vi "MainProgram.vi"() -> ()   [LabVIEW 2018]
uses:
  GitLabRepo/testers_labview/Library/Colas/FGV Control App Station.ctl
  GitLabRepo/testers_labview/ControlsApps/QueueLastState.ctl
  GitLabRepo/testers_labview/ControlsApps/ActionFGVConfig.ctl
  GitLabRepo/testers_labview/Library/NI/AMC_Klagan/Read Termination Message.vi
  GitLabRepo/testers_labview/Library/NI/AMC_Klagan/Create Single Message.vi
  GitLabRepo/testers_labview/Library/NI/AMC_Klagan/Update Message Routing Info.vi
  GitLabRepo/testers_labview/Library/NI/AMC_Klagan/Send Message.vi
  GitLabRepo/testers_labview/Library/NI/AMC_Klagan/Globals.vi
  GitLabRepo/testers_labview/Library/NI/AMC_Klagan/Queue Registry.vi
  <vilib>/Utility/file.llb/Write Delimited Spreadsheet (DBL).vi
  GitLabRepo/testers_labview/Library/NI/AMC_Klagan/AMC_Klagan.lvlib
panel:
  in  "ReadAnalogInputs":bool
  out "Out 7":bool
  out "Out 6":bool
  out "Out 5":bool
  out "Out 4":bool
  out "Out 3":bool
  out "Out 2":bool
  in  "WU_CreateUser":bool
  in  "WU_EditUser":bool
  in  "WU_RemoveUser":bool
  in  "WU_Role":enum16{"Manager", "Technician", "Operator"}(ring)=enum."Operator" caption="Role"
  in  "error in":errorcluster
  in  "Window":string
  # "ARDUINO UNO"
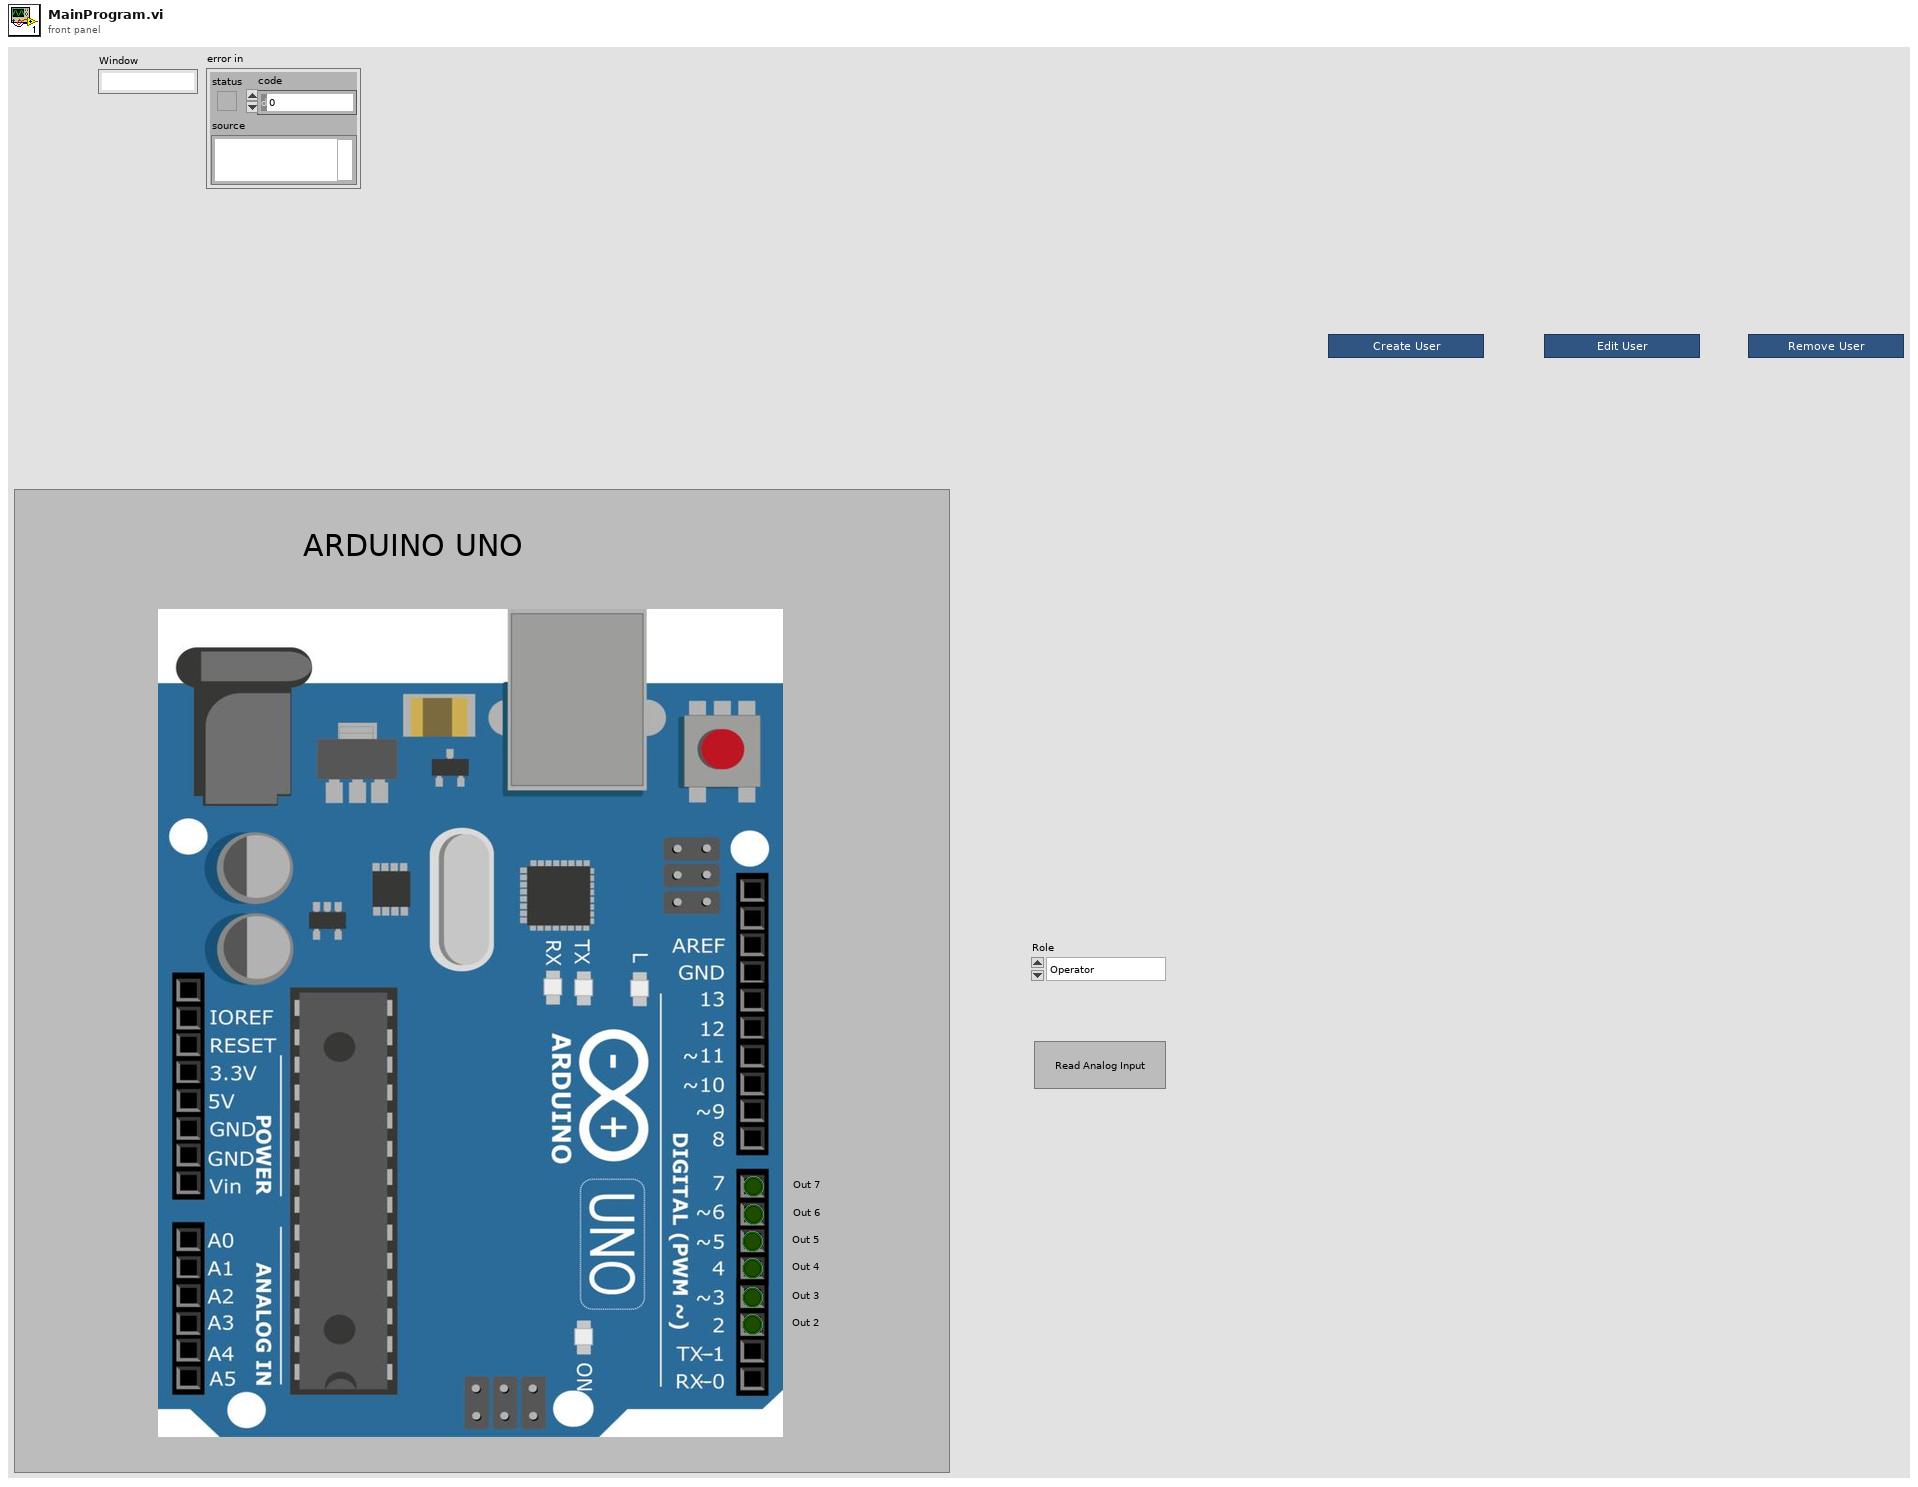
[diagram p1: front panel]
types:
  T1 = typedef "QueueLastState.ctl" = cluster{"LastState":string, "Data":variant}
  T2 = typedef "FGV Control App Station.ctl" = enum16{"Set", "Get All", "RemoveQueue", "Init"}
  T3 = typedef "AMC_Klagan.lvlib/Message Queue.ctl" = refnum<queue>
  T4 = typedef "ActionFGVConfig.ctl" = enum16{"SaveConfig", "ReadConfig"}
  T5 = typedef "GeneralConfig.ctl" = cluster{"General":path, "Path_Plataforma":path, "Path_Save_Sequences":path, "Path_Debugger":path, "Path_Logs_Tests":path, "Path_Reports":path, "Name_Station":string, "Path_Tests":path, "Path_Icons":path, "NumberOfCells":u32, "Path_TemplateReport":path, "Path_PowerUp":path, "Path_PowerDown":path, "Path_Abort":path, "Path_StartSequence":path, "Path_FinisSequence":path, "PortServerAPP":u32, "Path_Logs_App":path, "ExecutionDefSeqWhenOpen":bool, "LoadDefSeqWhenOpen":bool, "DefaultSequences":T6, "EnableSaveReports":bool, "EnableLogSequence":bool, "EnableDebuggerFile":bool, "Path_DefaultSequenceStart":path, "Path_DefaultSequenceAbort":path, "ManagerCommunication":T7, "Path_Factory":path, "Path_Variant":path, "Path_Model":path, "Path_SaveConfig":path, "SelectINI":string, "Path_ConfigPinOut":path, "Path_FailSequence":path, "Path_FinishExecutionSequence":path, "Path_DefaultSeqPowerUp":path, "Path_DefaultSeqPowerDown":path, "Path_DefaultSeqFinish":path, "Path_DefaultSeqFail":path, "Path_DefaultFinishExecution":path, "EnablePowerUpWhenOpen":bool, "EnablePowerDownWhenClose":bool, "EnableFinishExecution":bool, "SimultaneousStartCell":bool, "DefaultSimultaneousStartCellExecuteContinuously":bool, "DefaultHiddenStartSeq":bool, "DefaultHiddenAbortSeq":bool, "DefaultHiddenFinishExec":bool, "DefaultHiddenFailSeq":bool, "DefaultHiddenFinishSeq":bool, "DefaultHiddenPowerDown":bool, "DefaultHiddenPowerUp":bool, "Path_Users":path, "Path_File_Translate":path, "Path Icon 1":path, "Path Icon 2":path, "Path Image Login":path, "Check PCName Vs StationName":bool, "Windows Cells Layout":string, "Only One Test Plan for all cells":bool}
  T6 = typedef "DefaultSequncesLoad.ctl" = cluster{"Path_DefaultSeqCell 1":path, "Path_DefaultSeqCell 2":path, "Path_DefaultSeqCell 3":path, "Path_DefaultSeqCell 4":path, "Path_DefaultSeqCell 5":path, "Path_DefaultSeqCell 6":path, "Path_DefaultSeqCell 7":path, "Path_DefaultSeqCell 8":path, "Path_DefaultSeqCell 9":path}
  T7 = typedef "ConfiManagerCommunication.ctl" = cluster{"PortManComm":u32, "IPManager":string, "EnableManCom":bool}
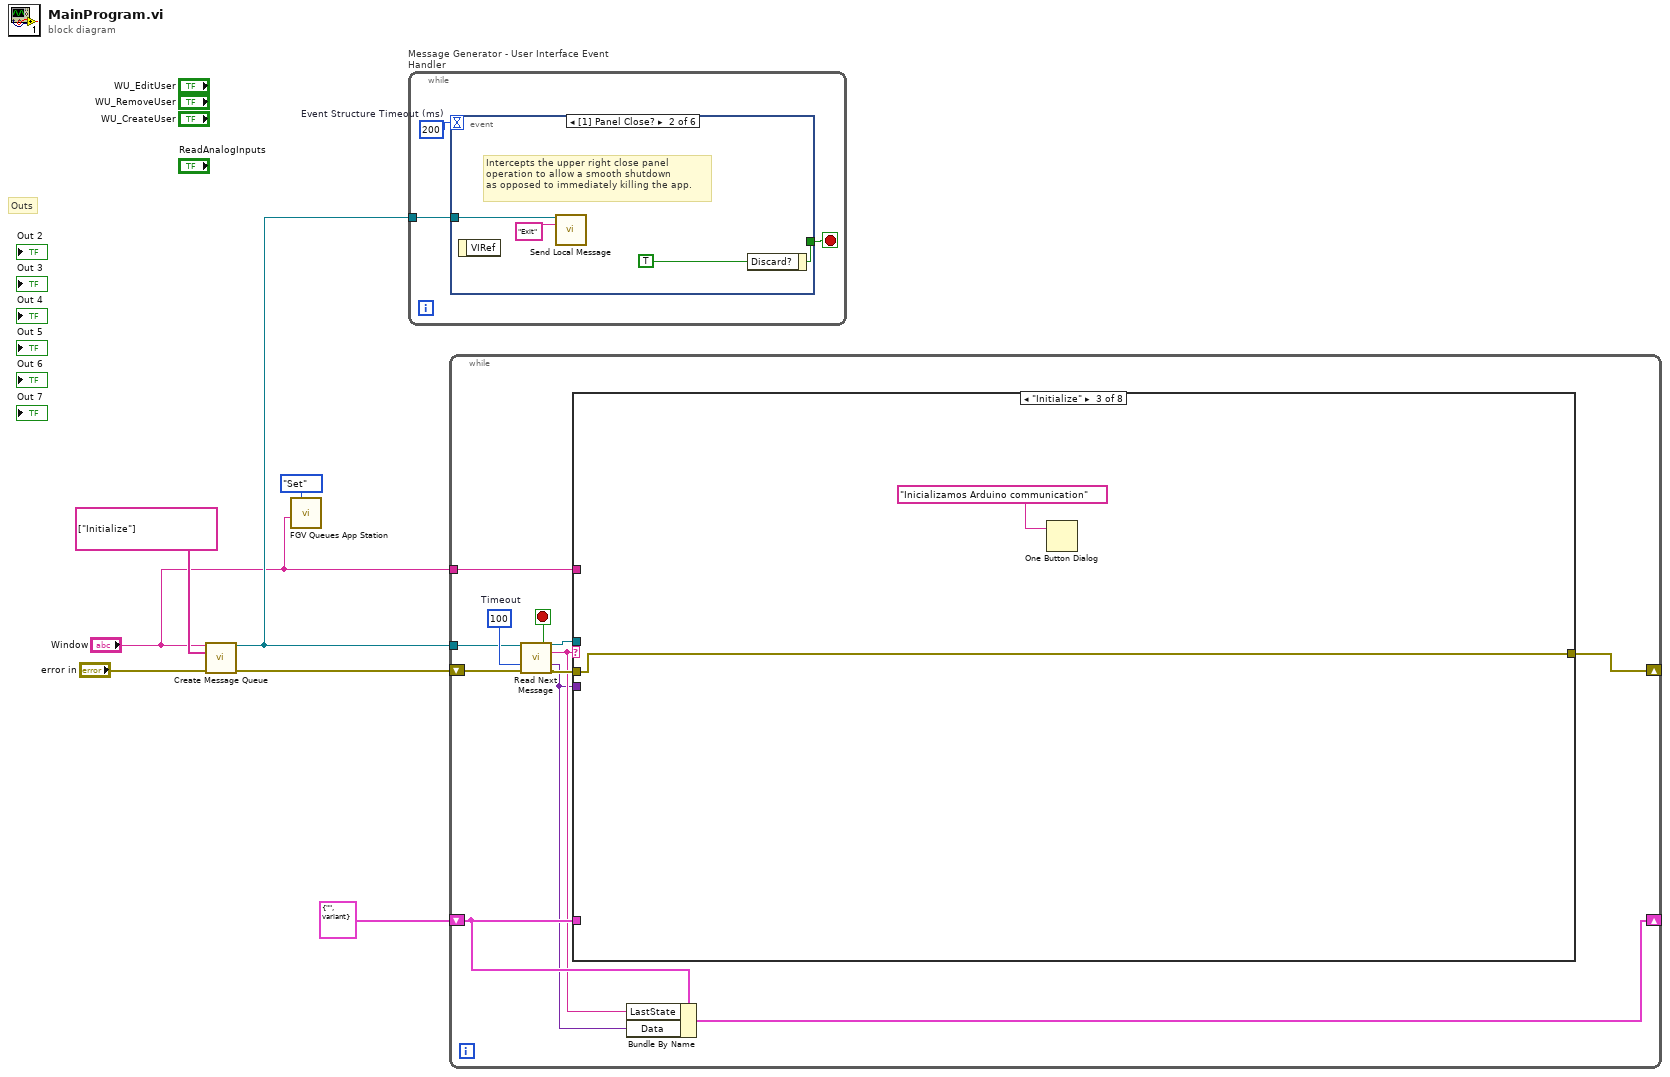
[diagram p0: block diagram]
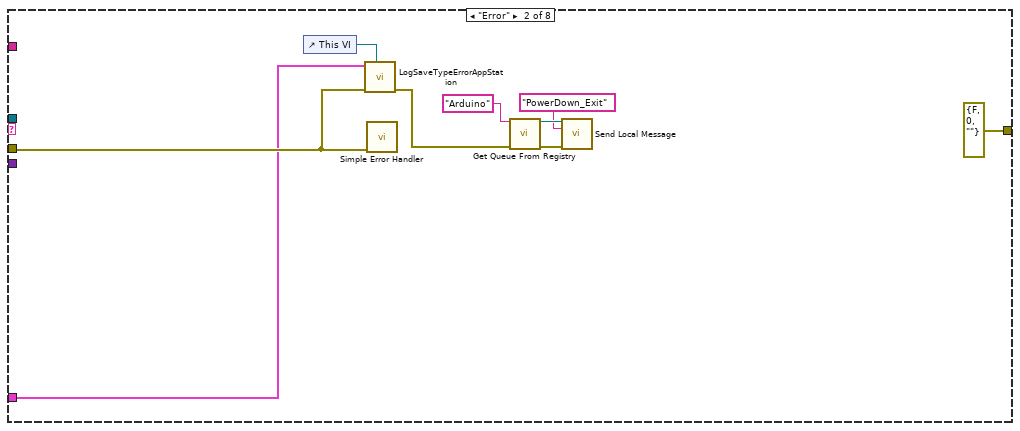
[diagram p3: hidden frame]
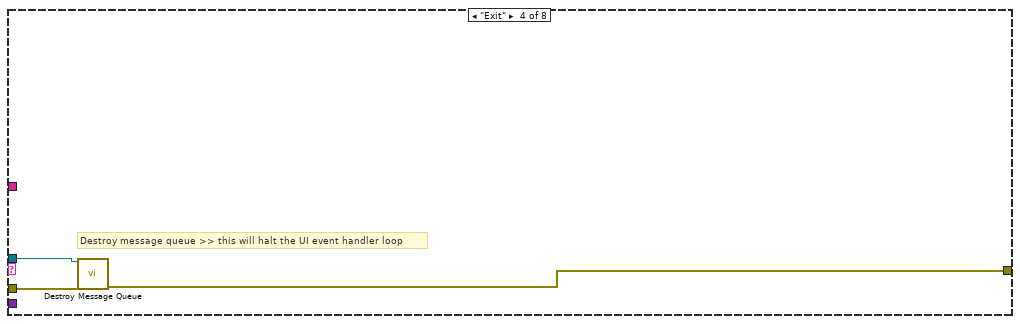
[diagram p4: hidden frame]
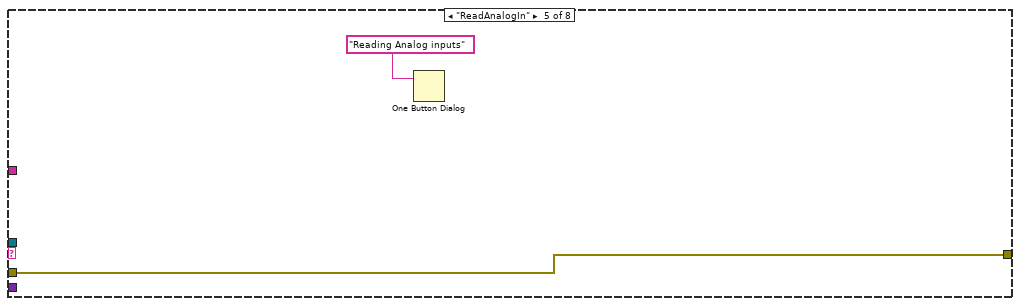
[diagram p5: hidden frame]
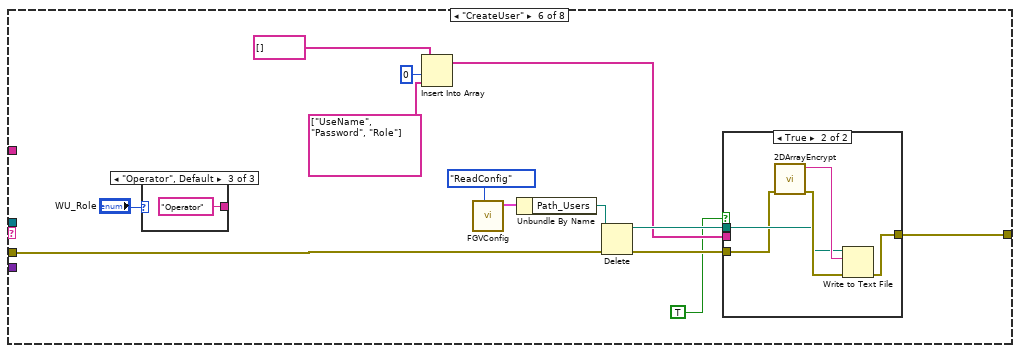
[diagram p6: hidden frame]
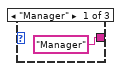
[diagram p7: hidden frame]
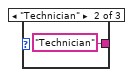
[diagram p8: hidden frame]
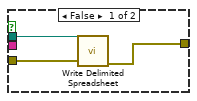
[diagram p9: hidden frame]
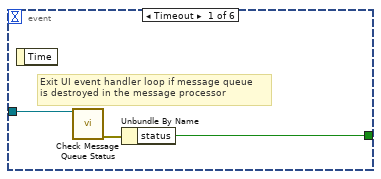
[diagram p12: hidden frame]
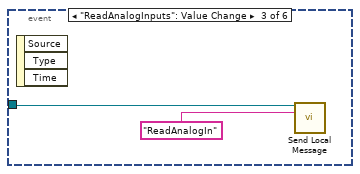
[diagram p13: hidden frame]
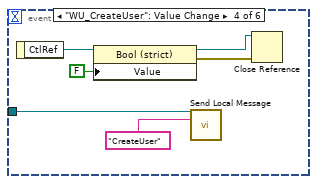
[diagram p14: hidden frame]
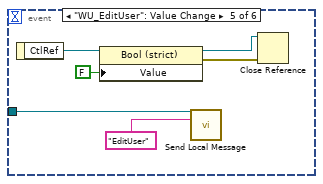
[diagram p15: hidden frame]
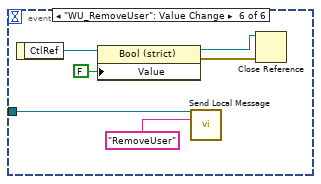
[diagram p16: hidden frame]
diagram:
  # "Outs"
  n1 = call "Create Message Queue.vi"("message queue name"="Window", "initial message names"=string[] ["Initialize"], "error in"="error in") -> ("message queue out"=w4:T3, "error out"=w3:errorcluster)  [unwired: 11 in]
  n2 = call "FGV Queues App Station.vi"("Control"=FGV_Control_App_Station."Set", "NameQueue"="Window") -> ()  [unwired: 7 in, 3 out]
  n3 = while "Message Generator - User Interface Event Handler" {
    tunnel: w4 -> [w8]
    stop <- w9 stop-if-true
    w10 = 200  # Event Structure Timeout (ms)
    n4 = event shown="[1] Panel Close?" {
      selector: _ -> [_ _ _ _ _ _]
      dyn-events: _ -> [_ _ _ _ _ _]
      timeout: w10 -> [_ _ _ _ _ _]
      tunnel: [w11 w16 _ _ _ _] -> w9
      tunnel: w8 -> [w12 w14 w17 w23 w29 w35]
      event Timeout {
        # "Exit UI event handler loop if message queue\nis destroyed in the message processor"
        n5 = event-data() -> ()  [unwired: 2 out]
        n6 = call "Check Message Queue Status.vi"("message queue in"=w12) -> ("error out"=w13:errorcluster)  [unwired: 10 in, 4 out]
        n7 = Unbundle By Name(w13) -> ("status"=w11:bool)
      }
      event Panel Close? {
        w16 = TRUE ("Discard?")
        # "Intercepts the upper right close panel\noperation to allow a smooth shutdown\nas opposed to immediately killing the app."
        n8 = event-data() -> ()  [unwired: 2 out]
        n9 = call "Send Local Message.vi"("message queue in"=w14, "message name"="Exit") -> ()  [unwired: 11 in, 3 out]
        n10 = event-data("Discard?"=w16) -> ()  [unwired: 1 in, 1 out]
      }
      event "ReadAnalogInputs": Value Change {
        n11 = event-data() -> ()  [unwired: 4 out]
        n12 = call "Send Local Message.vi"("message queue in"=w17, "message name"="ReadAnalogIn") -> ()  [unwired: 11 in, 3 out]
      }
      event "WU_CreateUser": Value Change {
        n13 = event-data() -> ("CtlRef"=w22:refnum<vi>)  [unwired: 1 out]
        n14 = property class="Bool (strict)"(reference=w22, "Value"=FALSE) -> (reference out=w19:refnum<vi>, error out=w20:errorcluster)  [unwired: 1 in]
        n15 = call "Send Local Message.vi"("message queue in"=w23, "message name"="CreateUser") -> ()  [unwired: 11 in, 3 out]
        n16 = Close Reference(reference=w19, error in (no error)=w20) -> ()  [unwired: 1 out]
      }
      event "WU_EditUser": Value Change {
        n17 = event-data() -> ("CtlRef"=w25:refnum<vi>)  [unwired: 1 out]
        n18 = property class="Bool (strict)"(reference=w25, "Value"=FALSE) -> (reference out=w26:refnum<vi>, error out=w27:errorcluster)  [unwired: 1 in]
        n19 = call "Send Local Message.vi"("message queue in"=w29, "message name"="EditUser") -> ()  [unwired: 11 in, 3 out]
        n20 = Close Reference(reference=w26, error in (no error)=w27) -> ()  [unwired: 1 out]
      }
      event "WU_RemoveUser": Value Change {
        n21 = event-data() -> ("CtlRef"=w31:refnum<vi>)  [unwired: 1 out]
        n22 = property class="Bool (strict)"(reference=w31, "Value"=FALSE) -> (reference out=w32:refnum<vi>, error out=w33:errorcluster)  [unwired: 1 in]
        n23 = call "Send Local Message.vi"("message queue in"=w35, "message name"="RemoveUser") -> ()  [unwired: 11 in, 3 out]
        n24 = Close Reference(reference=w32, error in (no error)=w33) -> ()  [unwired: 1 out]
      }
    }
  }
  n25 = while {
    tunnel: w4 -> [w44]
    tunnel: "Window" -> [w43]
    shift-right: [w42] -> _
    shift-left: w3 -> [w47]
    shift-right: [w41] -> _
    shift-left: T1 {"LastState"="", "Data"=variant} -> [w40]
    stop <- w46 stop-if-true
    w48 = 100  # Timeout
    n26 = call "Read Next Message.vi"("message queue in"=w44, "timeout (1 ms)"=w48, "error in"=w47) -> ("exit process?"=w46:bool, "message queue out"=w38:T3, "message name"=w39:string, "Variant"=w37:variant, "error out"=w45:errorcluster)  [unwired: 4 in, 4 out]
    n27 = case shown="\"Initialize\"" w39 {
      tunnel: w45 -> [w49 w51 w59 w63 w64 w73 w90 w91]
      tunnel: w43 -> [_ _ _ _ _ _ _ _]
      tunnel: [w49 errorcluster {"status"=FALSE, "code"=0, "source"=""} ("error out") w59 w62 w64 w72 w90 w91] -> w42
      tunnel: w40 -> [_ w50 _ _ _ _ _ _]
      tunnel: w38 -> [_ _ _ w61 _ _ _ _]
      tunnel: w37 -> [_ _ _ _ _ _ _ _]
      frame "", "Idle", Default {
      }
      frame "Error" {
        n28 = control-ref of="This VI"() -> (w53:refnum<vi>)
        n29 = call "LogSaveTypeErrorAppStation.vi"("reference"=w53, "error in (no error)"=w51, "Cluster"=w50) -> ("error out"=w58:errorcluster)  [unwired: 8 in]
        n30 = call <vilib>:"Simple Error Handler.vi"("error in (no error)"=w51) -> ()  [unwired: 1 in, 8 out]
        n31 = call "Get Queue From Registry.vi"("name"="Arduino" ("message queue name"), "error in"=w58) -> ("queue out"=w56:T3, "error out"=w57:errorcluster)  [unwired: 12 in]
        n32 = call "Send Local Message.vi"("message queue in"=w56, "message name"="PowerDown_Exit", "error in"=w57) -> ()  [unwired: 10 in, 3 out]
      }
      frame "Initialize" {
        n33 = One Button Dialog(message="Inicializamos Arduino communication") -> ()  [unwired: 1 in, 1 out]
      }
      frame "Exit" {
        # "Destroy message queue >> this will halt the UI event handler loop"
        n34 = call "Destroy Message Queue.vi"("message queue in"=w61, "error in"=w63) -> ("error out"=w62:errorcluster)  [unwired: 11 in, 2 out]
      }
      frame "ReadAnalogIn" {
        n35 = One Button Dialog(message="Reading Analog inputs") -> ()  [unwired: 1 in, 1 out]
      }
      frame "CreateUser" {
        n36 = case shown="\"Operator\", Default" "WU_Role" {
          tunnel: ["Manager" ("Password") "Technician" ("Password") "Operator" ("Password")] -> _
          frame "Manager" {
          }
          frame "Technician" {
          }
          frame "Operator", Default {
          }
        }
        n37 = Insert Into Array(array=string[] [], index=0 ("index (row)"), new element=string[] ["UseName", "Password", "Role"] ("new element/subarray")) -> (w70:string[])
        n38 = call "FGVConfig.vi"("ActionFGV"=ActionFGVConfig."ReadConfig") -> ("OutConfig"=w78:T5)  [unwired: 10 in]
        n39 = Unbundle By Name(w78) -> ("Path_Users"=w74:path)
        n40 = Delete(path (use dialog)=w74, error in=w73) -> (deleted path=w75:path, error out=w76:errorcluster)  [unwired: 3 in, 1 out]
        n41 = case shown="True" TRUE {
          tunnel: w76 -> [w84 w86]
          tunnel: w75 -> [w83 w87]
          tunnel: [w82 w85] -> w72
          tunnel: w70 -> [_ _]
          frame False {
            n42 = call-poly <vilib>:"Write Delimited Spreadsheet.vi"("file path (dialog if empty)"=w83, "error in (no error)"=w84) -> ("error out"=w82:errorcluster)  [unwired: 12 in, 1 out]
          }
          frame True {
            n43 = call "2DArrayEncrypt.vi"("error in (no error)"=w86) -> ("error out"=w88:errorcluster, "Output text"=w89:string)  [unwired: 9 in]
            n44 = Write to Text File(file (use dialog)=w87, text=w89, error in=w88) -> (error out=w85:errorcluster)  [unwired: 1 in, 2 out]
          }
        }
      }
      frame "EditUser" {
      }
      frame "RemoveUser" {
      }
    }
    n45 = Bundle By Name(cluster=w40, "LastState"=w39, "Data"=w37) -> (w41:T1)
  }
